vi "Initialize Menu Items.vi"(8 "error in (no error)":errorcluster, 10 "Config":T1, 11 "Menu Ref":refnum<k9>) -> (0 "error out":errorcluster)   [LabVIEW 2020, in "VI Properties Editor.lvlib"]
doc: "Initializes several menu items related to options and recently viewed folders/files in <B>Config</B>."
uses:
  VI Properties Editor.lvlib
  CTLs/Config.ctl
  CTLs/Filter Info.ctl
  CTLs/Filter Column.ctl
  CTLs/Filter Type.ctl
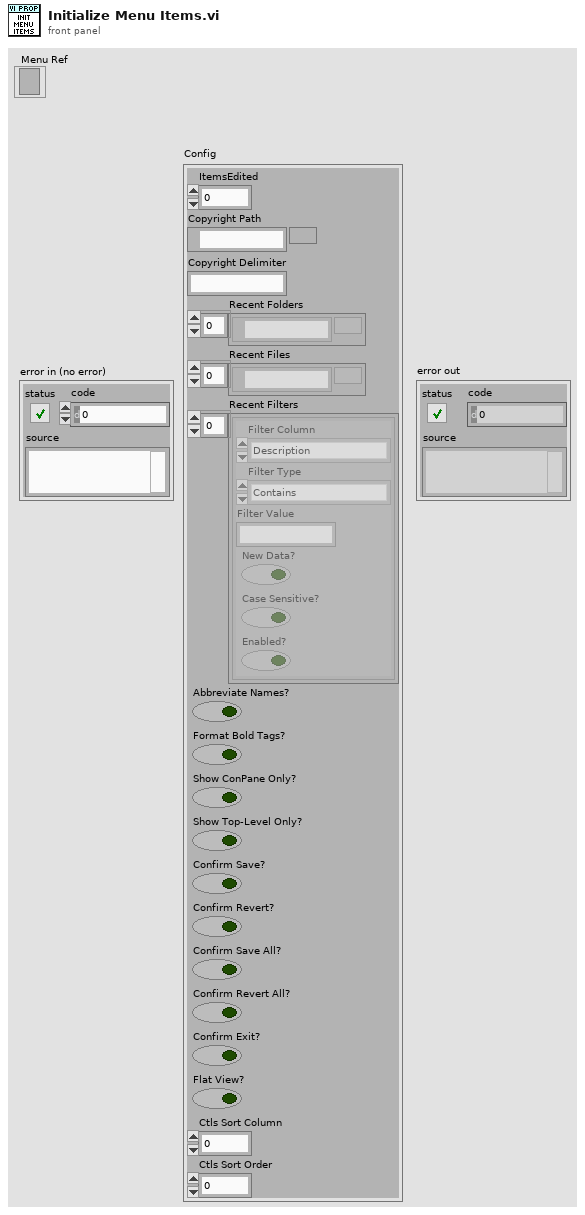
[diagram p1: front panel]
types:
  T1 = typedef "VI Properties Editor.lvlib/Config.ctl" = cluster{"ItemsEdited":u32, "Copyright Path":path, "Copyright Delimiter":string, "Recent Folders":path[], "Recent Files":path[], "Recent Filters":T2[], "Abbreviate Names?":bool, "Format Bold Tags?":bool, "Show ConPane Only?":bool, "Show Top-Level Only?":bool, "Confirm Save?":bool, "Confirm Revert?":bool, "Confirm Save All?":bool, "Confirm Revert All?":bool, "Confirm Exit?":bool, "Flat View?":bool, "Ctls Sort Column":i32, "Ctls Sort Order":i32}
  T2 = typedef "VI Properties Editor.lvlib/Filter Info.ctl" = cluster{"Filter Column":T3, "Filter Type":T4, "Filter Value":string, "New Data?":bool, "Case Sensitive?":bool, "Enabled?":bool}
  T3 = typedef "VI Properties Editor.lvlib/Filter Column.ctl" = enum16{"Name", "Path", "Type", "Window Title", "Description", "Help Path", "Help Tag", "Custom Title?", "Reentrancy", "Inlined?", "Help URL", "Help Type", "Allow Debugging?", "Auto Error Handling?", "Run When Opened?", "Suspend When Called?", "Priority", "Preferred Exec Sytem", "Control Label", "Control Caption", "Control Description", "Control Tip Strip"}
  T4 = typedef "VI Properties Editor.lvlib/Filter Type.ctl" = enum16{"Contains", "Equals", "Starts with", "Ends with", "Is empty", "Does not contain", "Does not equal", "Is not empty"}
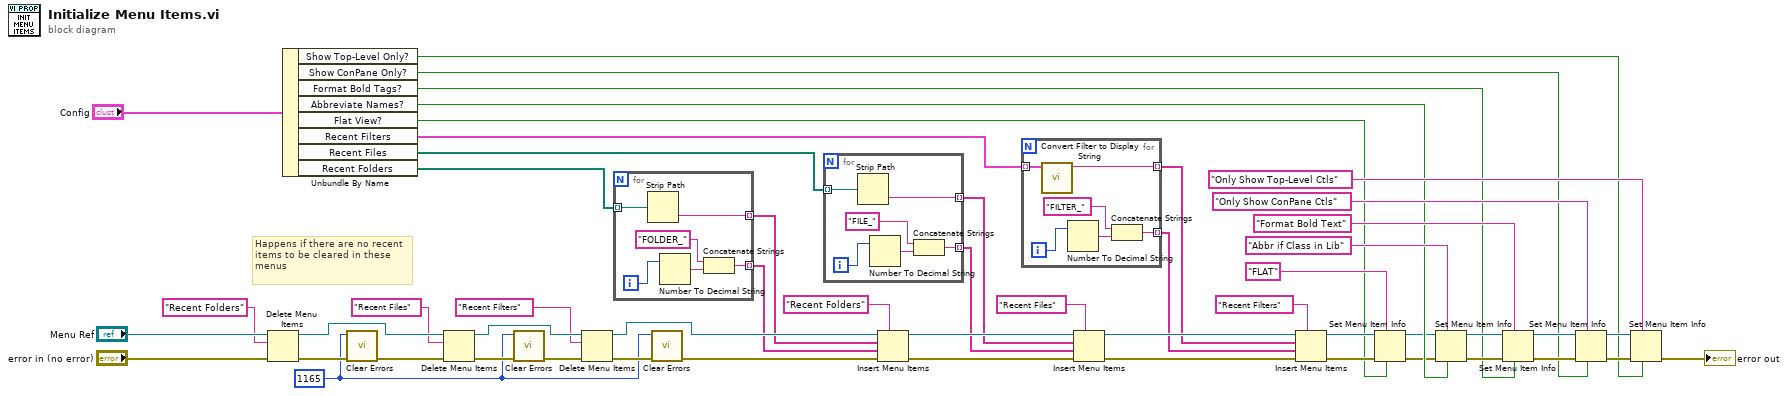
[diagram p0: block diagram]
diagram:
  w9 = 1165
  # "Happens if there are no recent items to be cleared in these menus"
  n1 = Delete Menu Items(6:"error in (no error)", 8:"Recent Folders" ("menu tag"), 9:"Menu Ref") -> (0:w27:errorcluster, 3:w49:refnum<k9>)  [unwired: 1 in]
  n2 = Unbundle By Name("Config") -> ("Show Top-Level Only?"=w1:bool, "Show ConPane Only?"=w20:bool, "Format Bold Tags?"=w29:bool, "Abbreviate Names?"=w30:bool, "Flat View?"=w4:bool, "Recent Filters"=w19:T2[], "Recent Files"=w33:path[], "Recent Folders"=w39:path[])
  n3 = call <vilib>:"Clear Errors.vi"("error in (no error)"=w27, "specific error code to clear (0: all)"=w9) -> ("error out"=w22:errorcluster)  [unwired: 4 in, 1 out]
  n4 = Delete Menu Items(6:w22, 8:"Recent Files" ("menu tag"), 9:w49) -> (0:w28:errorcluster, 3:w12:refnum<k9>)  [unwired: 1 in]
  n5 = call <vilib>:"Clear Errors.vi"("error in (no error)"=w28, "specific error code to clear (0: all)"=w9) -> ("error out"=w23:errorcluster)  [unwired: 4 in, 1 out]
  n6 = Delete Menu Items(6:w23, 8:"Recent Filters" ("menu tag"), 9:w12) -> (0:w13:errorcluster, 3:w51:refnum<k9>)  [unwired: 1 in]
  n7 = for {
    tunnel: w39 -> [w58] mode=indexing
    tunnel: [w55] -> w34 mode=indexing
    tunnel: [w54] -> w35 mode=indexing
    i -> [w59]
    n8 = Strip Path(path=w58) -> (name=w54:string)  [unwired: 1 out]
    n9 = Number To Decimal String(number=w59) -> (decimal integer string=w57:string)  [unwired: 1 in]
    n10 = Concatenate Strings("FOLDER_", w57) -> (w55:string)
  }
  n11 = call <vilib>:"Clear Errors.vi"("error in (no error)"=w13, "specific error code to clear (0: all)"=w9) -> ("error out"=w10:errorcluster)  [unwired: 4 in, 1 out]
  n12 = for {
    tunnel: w33 -> [w64] mode=indexing
    tunnel: [w61] -> w32 mode=indexing
    tunnel: [w60] -> w31 mode=indexing
    i -> [w65]
    n13 = Strip Path(path=w64) -> (name=w60:string)  [unwired: 1 out]
    n14 = Number To Decimal String(number=w65) -> (decimal integer string=w63:string)  [unwired: 1 in]
    n15 = Concatenate Strings("FILE_", w63) -> (w61:string)
  }
  n16 = Insert Menu Items(5:"Recent Folders" ("menu tag"), 6:w10, 7:w34, 8:w35, 9:w51) -> (0:w45:errorcluster, 3:w36:refnum<k9>)  [unwired: 1 in, 1 out]
  n17 = for {
    tunnel: [w68] -> w15 mode=indexing
    tunnel: w19 -> [w67] mode=indexing
    tunnel: [w66] -> w14 mode=indexing
    i -> [w71]
    n18 = call "Convert Filter to Display String.vi"("Filter Info"=w67) -> ("String"=w66:string)  [unwired: 10 in]
    n19 = Number To Decimal String(number=w71) -> (decimal integer string=w70:string)  [unwired: 1 in]
    n20 = Concatenate Strings("FILTER_", w70) -> (w68:string)
  }
  n21 = Insert Menu Items(5:"Recent Files" ("menu tag"), 6:w45, 7:w32, 8:w31, 9:w36) -> (0:w44:errorcluster, 3:w17:refnum<k9>)  [unwired: 1 in, 1 out]
  n22 = Insert Menu Items(5:"Recent Filters" ("menu tag"), 6:w44, 7:w15, 8:w14, 9:w17) -> (0:w18:errorcluster, 3:w7:refnum<k9>)  [unwired: 1 in, 1 out]
  n23 = Set Menu Item Info(6:w4, 7:"FLAT" ("item tag"), 8:w18, 11:w7) -> (0:w8:errorcluster, 3:w6:refnum<k9>)  [unwired: 3 in]
  n24 = Set Menu Item Info(6:w30, 7:"Abbr if Class in Lib" ("menu tag"), 8:w8, 11:w6) -> (0:w48:errorcluster, 3:w41:refnum<k9>)  [unwired: 3 in]
  n25 = Set Menu Item Info(6:w29, 7:"Format Bold Text" ("item tag"), 8:w48, 11:w41) -> (0:w47:errorcluster, 3:w21:refnum<k9>)  [unwired: 3 in]
  n26 = Set Menu Item Info(6:w20, 7:"Only Show ConPane Ctls" ("item tag"), 8:w47, 11:w21) -> (0:w3:errorcluster, 3:w53:refnum<k9>)  [unwired: 3 in]
  n27 = Set Menu Item Info(6:w1, 7:"Only Show Top-Level Ctls" ("item tag"), 8:w3, 11:w53) -> (0:→"error out":errorcluster)  [unwired: 3 in, 1 out]
